vi "EndTestSuite.vi"(8 "error in (no error)":errorcluster, 10 "TestSuite":refnum<class "TestSuite.lvclass">, 11 "ResultTreeListener in":refnum<class "ResultTreeListener.lvclass">) -> (0 "error out":errorcluster, 3 "ResultTreeListener out":refnum<class "ResultTreeListener.lvclass">)   [LabVIEW 2019, in "ResultTreeListener.lvclass"]
doc: "A test suite ended."
uses:
  ResultTreeListener.lvclass
  TestSuite/TestSuite.lvclass
  ResultTreeListener.lvclass/ResultTreeListener.ctl
  ResultTree/Icon.ctl
  ResultTree/ResultTree.lvclass
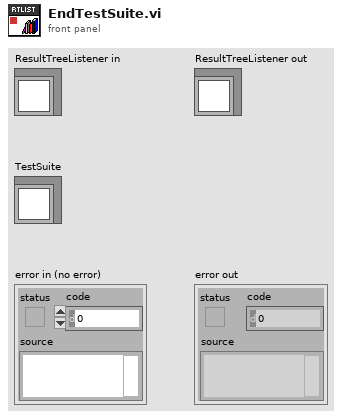
[diagram p1: front panel]
types:
  T1 = typedef "ResultTree.lvclass/Icon.ctl" = enum16{"None", "Passed", "Failed", "Error"}
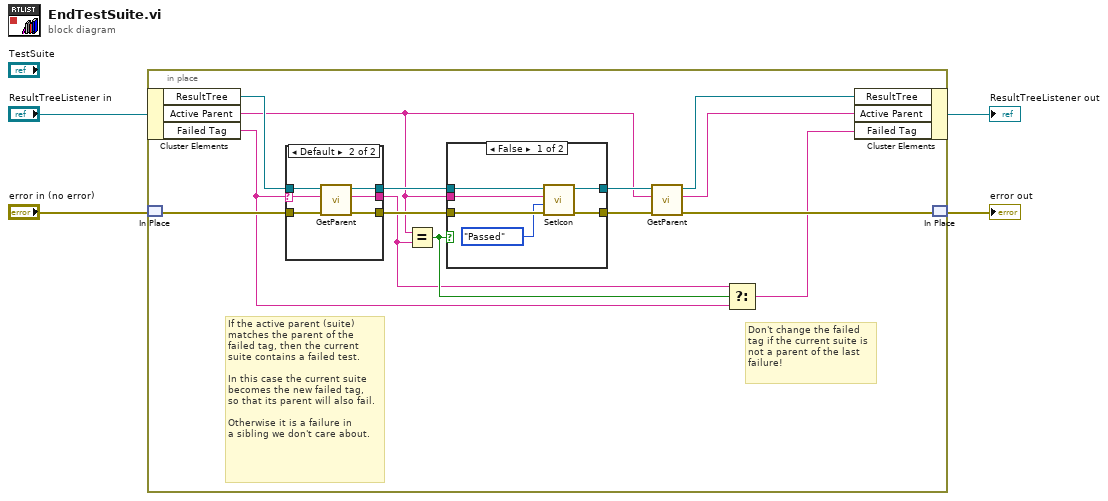
[diagram p0: block diagram]
diagram:
  n1 = in-place {
    # "Don't change the failed\ntag if the current suite is\nnot a parent of the last\nfailure!"
    # "If the active parent (suite)\nmatches the parent of the\nfailed tag, then the current\nsuite contains a failed test.\n\nIn this case the current suite\nbecomes the new failed tag,\nso that its parent will also fail.\n\nOtherwise it is a failure in\na sibling we don't care about."
    n2 = in-place-cluster #1("ResultTreeListener in") -> ("ResultTree"=w11:refnum<class "ResultTree.lvclass">, "Active Parent"=w7:string, "Failed Tag"=w6:string)
    n3 = in-place-match #2("error in (no error)") -> (w13:errorcluster)
    n4 = case shown="Default" w6 {
      selector: w6 -> [_ w29]
      tunnel: w13 -> [w27 w34]
      tunnel: [w27 w33] -> w12
      tunnel: w11 -> [w28 w32]
      tunnel: [w28 w31] -> w10
      tunnel: [_ w30] -> w5
      frame "" {
      }
      frame Default {
        n5 = call "GetParent.vi"("error in (no error)"=w34, "Tag"=w29, "ResultTree in"=w32) -> ("error out"=w33:errorcluster, "Parent Tag"=w30:string, "ResultTree out"=w31:refnum<class "ResultTree.lvclass">)  [unwired: 6 in]
      }
    }
    n6 = Equal?(x=w7, y=w5) -> (x = y?=w9:bool)
    n7 = case shown="False" w9 {
      tunnel: w12 -> [w24 w25]
      tunnel: [w23 w25] -> w16
      tunnel: w10 -> [w22 w26]
      tunnel: [w21 w26] -> w15
      tunnel: w7 -> [w20 _]
      frame False {
        n8 = call "SetIcon.vi"("error in (no error)"=w24, "Icon"=Icon."Passed", "Tag Name"=w20, "ResultTree in"=w22) -> ("error out"=w23:errorcluster, "ResultTree out"=w21:refnum<class "ResultTree.lvclass">)  [unwired: 6 in]
      }
      frame True {
      }
    }
    n9 = call "GetParent.vi"("error in (no error)"=w16, "Tag"=w7, "ResultTree in"=w15) -> ("error out"=w17:errorcluster, "Parent Tag"=w14:string, "ResultTree out"=w18:refnum<class "ResultTree.lvclass">)  [unwired: 6 in]
    n10 = Select(t=w5, s=w9, f=w6) -> (s? t:f=w8:string)
    n11 = in-place-cluster #1("ResultTree"=w18, "Active Parent"=w14, "Failed Tag"=w8) -> (→"ResultTreeListener out":refnum<class "ResultTreeListener.lvclass">)
    n12 = in-place-match #2(w17) -> (→"error out":errorcluster)
  }
